vi "SS2 Live_Get Control Label & Settings Element.vi"(8 "Error In":errorcluster, 11 "CtlRef":refnum<vi>) -> (0 "Error Out":errorcluster, 1 "Control Label":string, 3 "Settings Element":T1)   [LabVIEW 2019]
uses:
  SS2 Live_Settings List.ctl
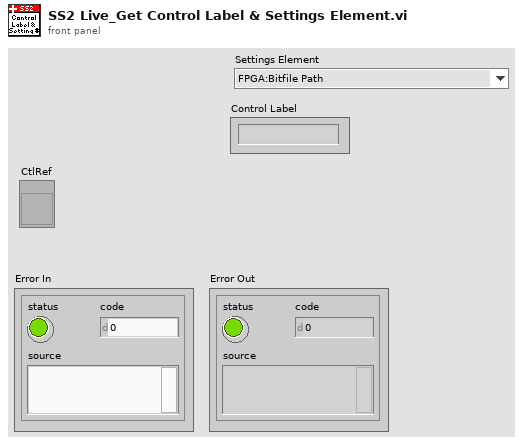
[diagram p1: front panel]
types:
  T1 = typedef "SS2 Live_Settings List.ctl" = enum16{"FPGA:Bitfile Path", "FPGA:Bitfile Version", "Acquisition Parameters:SS2 DAQ Parameters", "Acquisition Parameters:Gate Configuration Array", "Acquisition Parameters:Buffer Size (# Gates)", "File Information:File Information", "File Information:# Datasets in Series", "Image Parameters:Image ROI Information", "Image Parameters:Image Binning Options", "UI Parameters:Histogram Bins Number"}
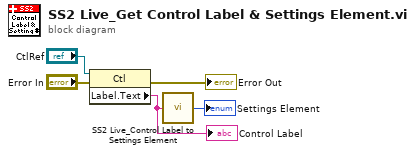
[diagram p0: block diagram]
diagram:
  n1 = property class="Ctl"(reference="CtlRef", error in="Error In") -> (error out=→"Error Out":errorcluster, "Label.Text"=w2:string)  [unwired: 1 out]
  "Control Label" <- w2
  n2 = call "SS2 Live_Control Label to Settings Element.vi"("Control Label"=w2) -> ("Settings List Element"=→"Settings Element":T1)  [unwired: 8 in]
